vi "Insert Custom Glyphs.vi"(8 "error in (no error)":errorcluster, 11 "File Explorer in":refnum<class "File Explorer.lvclass">) -> (0 "error out":errorcluster, 3 "File Explorer out":refnum<class "File Explorer.lvclass">)   [LabVIEW 2017, in "File Explorer.lvlib" / "File Explorer.lvclass"]
uses:
  <vilib>/gpm_packages/@cs/file-explorer-extension/Source/File Explorer/File Explorer/File Explorer.lvclass
  <vilib>/gpm_packages/@cs/file-explorer-extension/Source/File Explorer/File Explorer/File Explorer.lvclass/File Explorer.ctl
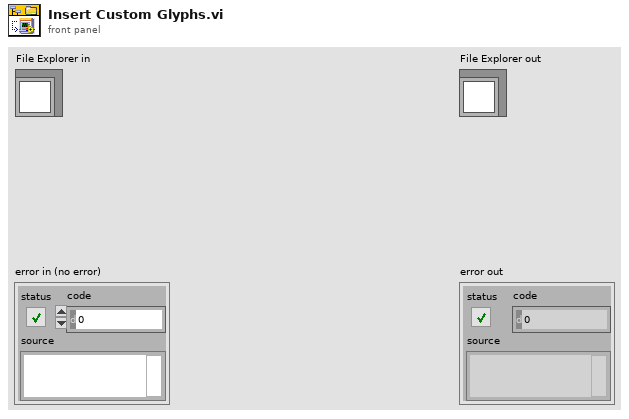
[diagram p1: front panel]
types:
  T1 = typedef "File Explorer.lvlib/File Explorer.lvclass/Custom Glyph Definition.ctl" = cluster{"Extension":string, "Glyph":T2}
  T2 = typedef "imagedata.ctl" = cluster{"image type":i32, "image depth":i32, "image":u8[], "mask":u8[], "colors":u32[], "Rectangle":cluster{"left":i16, "top":i16, "right":i16, "bottom":i16}}
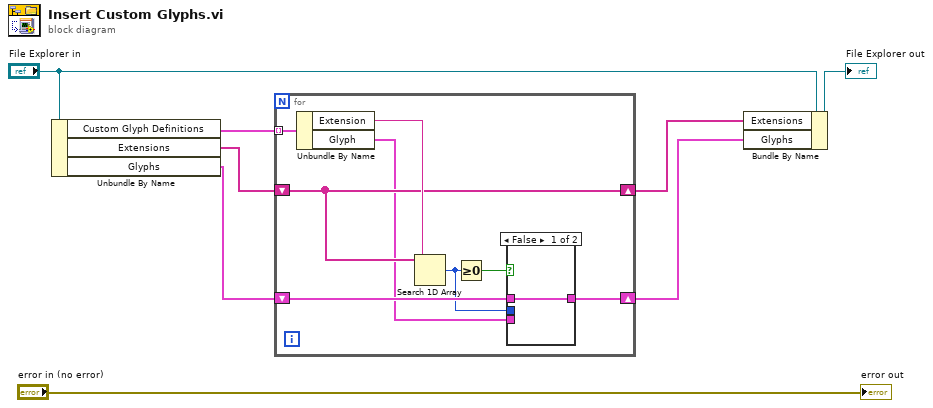
[diagram p0: block diagram]
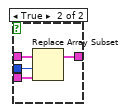
[diagram p2: hidden frame]
diagram:
  n1 = Unbundle By Name("File Explorer in") -> ("Custom Glyph Definitions"=w8:T1[], "Extensions"=w3:string[], "Glyphs"=w2:T2[])
  n2 = for {
    tunnel: w8 -> [w16] mode=indexing
    shift-right: [w13] -> w6
    shift-left: w2 -> [w14]
    shift-right: [w10] -> w7
    shift-left: w3 -> [w10]
    n3 = Unbundle By Name(w16) -> ("Extension"=w15:string, "Glyph"=w9:T2)
    n4 = Search 1D Array(1D array=w10, element=w15) -> (index of element=w11:i32)  [unwired: 1 in]
    n5 = Greater Or Equal To 0?(x=w11) -> (x >= 0?=w12:bool)
    n6 = case shown="False" w12 {
      tunnel: w14 -> [w17 w21]
      tunnel: [w17 w20] -> w13
      tunnel: w11 -> [_ w19]
      tunnel: w9 -> [_ w18]
      frame False {
      }
      frame True {
        n7 = Replace Array Subset(array=w21, new element=w18, index=w19) -> (w20:T2[])
      }
    }
  }
  n8 = Bundle By Name(cluster="File Explorer in", "Extensions"=w7, "Glyphs"=w6) -> (→"File Explorer out":refnum<class "File Explorer.lvclass">)
  "error out" <- "error in (no error)"
